vi "Initialize Network.vi"(8 "error in (no error)":errorcluster, 11 "msg cluster in":T1) -> (0 "error out":errorcluster, 2 "hardware controls out":T4={"force sensor channel"="", "servo task"="", "led task"="", "camera port"="", "cam freq (hz)"=30.0, "force freq (hz)"=30.0, "color pane"=0, "servo freq (hz)"=30.0} {"color pane" items=["Blue", "Red", "Green", "Saturation", "Value", "Intensity", "Luminance", "Hue", ""]}, 3 "msg cluster out":T1)   [LabVIEW 2020]
uses:
  Messaging Cluster.ctl
  Hardware/Sensors/Cameras/Camera.lvclass
  C:/Users/jharw/Documents/1 Folder to Rule them All/UMD/Inflation-Apparatus/src/Hardware/General Hardware.lvclass
  Hardware/Sensors/Force Sensors/Force Sensor.lvclass
  Hardware/Actuators/Servos/Servo.lvclass
  Hardware/Actuators/Switches/Switch.lvclass
  Inflation Test/Parameter Class/IA Test Parameters.lvclass
  Controllers/Controller.lvclass
  Controller Loop/Message and Data.ctl
  GUI/Main GUI Loop/Handler.ctl
  Inflation Test/Result Handling/Inflation Test Numeric Results.ctl
  Inflation Test/Controls/Hardware Options.ctl
  <vilib>/userdefined/High Color/IMAQdx.ctl
  Hardware/Sensors/Cameras/Simulated Camera/Simulated Camera.lvclass
  C:/Users/jharw/Documents/1 Folder to Rule them All/UMD/Inflation-Apparatus/src/Hardware/Sensors/Cameras/Camera.lvclass
  Hardware/Sensors/Force Sensors/Simulated Force Sensor/Simulated Force Sensor.lvclass
  C:/Users/jharw/Documents/1 Folder to Rule them All/UMD/Inflation-Apparatus/src/Hardware/Sensors/Force Sensors/Force Sensor.lvclass
  Hardware/Actuators/Servos/Simulated Servo/Simulated Servo.lvclass
  C:/Users/jharw/Documents/1 Folder to Rule them All/UMD/Inflation-Apparatus/src/Hardware/Actuators/Servos/Servo.lvclass
  Hardware/Actuators/Switches/Simulated Switch/Simulated Switch.lvclass
  C:/Users/jharw/Documents/1 Folder to Rule them All/UMD/Inflation-Apparatus/src/Hardware/Actuators/Switches/Switch.lvclass
  Hardware/General Hardware.lvclass/General Hardware.ctl
  Controllers/Simulated Controller/Simulated Controller.lvclass
  C:/Users/jharw/Documents/1 Folder to Rule them All/UMD/Inflation-Apparatus/src/Controllers/Controller.lvclass
  Controllers/PID/PID Controller.lvclass
  Controllers/PID/PID Controller.lvclass/PID Controller.ctl
  Hardware/General Hardware.lvclass
panel:
  in  "continue":bool
  in  "controller tab":enum32{"Simulated Controller", "PID Controller"}(tab)=enum."PID Controller"
  in  "PID gains":T6={"proportional gain (Kc)"=1.0, "integral time (Ti, min)"=0.01, "derivative time (Td, min)"=0.0} caption="PID GAINS" {"derivative time (Td, min)" format="%.3f"; "integral time (Ti, min)" format="%.3f"; "proportional gain (Kc)" format="%.3f"}
  in  "hardware tab":enum32{"Real Hardware", "Simulated Hardware"}(tab)
  in  "real hardware controls":T4={"force sensor channel"="", "servo task"="", "led task"="", "camera port"="", "cam freq (hz)"=30.0, "force freq (hz)"=30.0, "color pane"=0, "servo freq (hz)"=30.0} {"color pane" items=["Blue", "Red", "Green", "Saturation", "Value", "Intensity", "Luminance", "Hue", ""]}
  in  "sim servo freq (hz)":dbl=30.0
  in  "sim cam freq (hz)":dbl=30.0
  in  "sim force freq (hz)":dbl=30.0
  # "HARDWARE AND CONTROL INITIALIZATION"
  # "FORCE SENSOR CHANNEL"
  # "SERVO CHANNEL"
  # "LED CHANNEL"
  # "CAMERA PORT"
  # "CAMERA FREQUENCY (HZ):"
  # "FORCE FREQUENCY (HZ):"
  # "SERVO FREQUENCY (HZ):"
  # "COLOR PANE:"
  # "NO CONTROLLER WILL BE USED, GENERATED PULSES WILL BE RANDOM"
  # "FORCE SENSOR CHANNEL"
  # "SERVO CHANNEL"
  # "LED CHANNEL"
  # "CAMERA PORT"
  # "CAMERA FREQUENCY (HZ):"
  # "FORCE FREQUENCY (HZ):"
  # "SERVO FREQUENCY (HZ):"
  # "COLOR PANE:"
  # "CAMERA FREQUENCY (HZ):"
  # "FORCE FREQUENCY (HZ):"
  # "SERVO FREQUENCY (HZ):"
  # "CAMERA AND FORCE DATA GENERATED WILL BE RANDOMIZED\n\nSERVO AND LED WILL NOT INTERFACE WITH PHYSICAL HARDWARE"
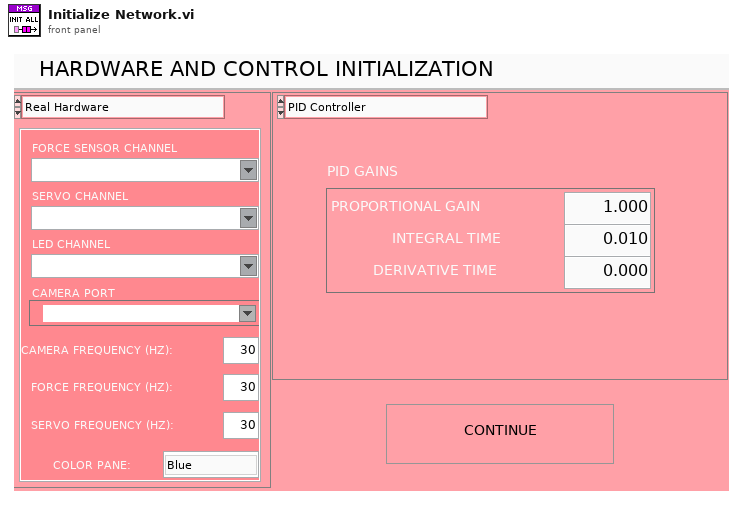
[diagram p1: front panel]
types:
  T1 = typedef "Messaging Cluster.ctl" = cluster{"cam queue":refnum<queue>, "fs queue":refnum<queue>, "servo queue":refnum<queue>, "switch queue":refnum<queue>, "cam class":refnum<class "Camera.lvclass">, "fs class":refnum<class "Force Sensor.lvclass">, "servo class":refnum<class "Servo.lvclass">, "switch class":refnum<class "Switch.lvclass">, "switch notifier":refnum<notifier>, "servo notifier":refnum<notifier>, "fs notifier":refnum<notifier>, "cam notifier":refnum<notifier>, "rgst evnt":refnum<event-registration>, "user event":refnum<user-event>, "ctlr queue":refnum<queue>, "main gui queue":refnum<queue>, "main gui type":T2, "cntlr type":T3, "gui notifier":refnum<notifier>, "ia test notifier":refnum<notifier>}
  T2 = typedef "Handler.ctl" = cluster{"bool ref":refnum<vi>, "error":errorcluster, "msg":string, "status":string}
  T3 = typedef "Message and Data.ctl" = cluster{"msg":string, "ia test param":refnum<class "IA Test Parameters.lvclass">, "controller type":refnum<class "Controller.lvclass">, "folder path":path, "file name":string, "file comments":string}
  T4 = typedef "Hardware Options.ctl" = cluster{"force sensor channel":tag, "servo task":tag, "led task":tag, "camera port":T5, "cam freq (hz)":dbl, "force freq (hz)":dbl, "color pane":i32, "servo freq (hz)":dbl}
  T5 = typedef "IMAQdx.ctl" = refnum<k21>
  T6 = cluster{"proportional gain (Kc)":dbl, "integral time (Ti, min)":dbl, "derivative time (Td, min)":dbl}
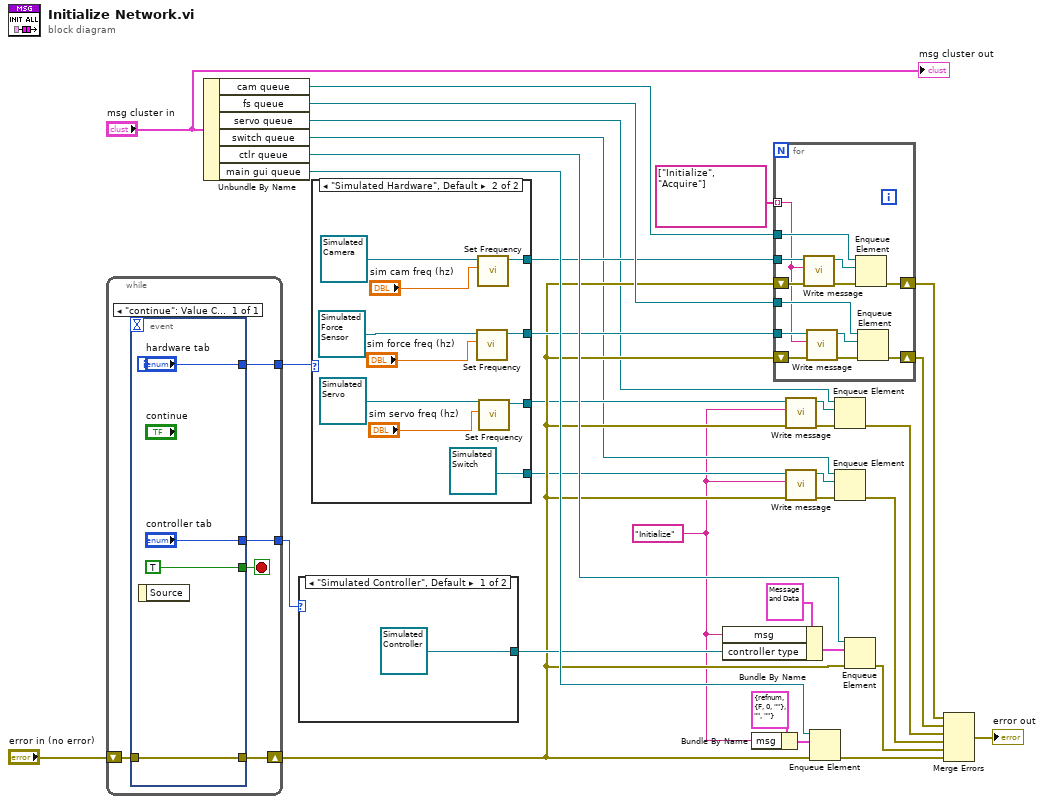
[diagram p0: block diagram]
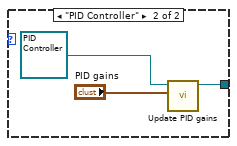
[diagram p2: hidden frame]
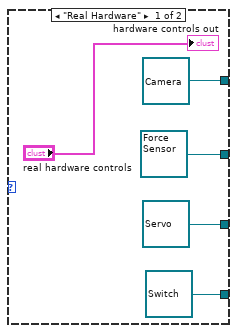
[diagram p3: hidden frame]
diagram:
  w4 = "Initialize" ("message")
  n1 = while {
    shift-right: [w37] -> w15
    shift-left: "error in (no error)" -> [w38]
    tunnel: [w35] -> w20
    tunnel: [w34] -> w17
    stop <- w36 stop-if-true
    n2 = event shown="[0] \"continue\": Value Change" {
      selector: _ -> [_]
      dyn-events: _ -> [_]
      timeout: _ -> [_]
      tunnel: w38 -> [w42]
      tunnel: [w42] -> w37
      tunnel: [TRUE] -> w36
      tunnel: ["hardware tab"] -> w35
      tunnel: ["controller tab"] -> w34
      event "continue": Value Change {
        n3 = event-data() -> ()  [unwired: 1 in, 1 out]
      }
    }
  }
  n4 = Unbundle By Name("msg cluster in") -> ("cam queue"=w3:refnum<queue>, "fs queue"=w32:refnum<queue>, "servo queue"=w9:refnum<queue>, "switch queue"=w8:refnum<queue>, "ctlr queue"=w31:refnum<queue>, "main gui queue"=w28:refnum<queue>)
  n5 = case shown="\"Simulated Controller\", Default" w17 {
    tunnel: [refnum<class "Simulated Controller.lvclass"> refnum ("Simulated Controller.lvclass") w44] -> w16
    frame "Simulated Controller", Default {
    }
    frame "PID Controller" {
      n6 = call "Update PID gains.vi"("PID gains"="PID gains", "PID Controller in"=refnum<class "PID Controller.lvclass"> refnum ("PID Controller.lvclass")) -> ("PID Controller out"=w44:refnum<class "PID Controller.lvclass">)  [unwired: 8 in, 1 out]
    }
  }
  n7 = case shown="\"Simulated Hardware\", Default" w20 {
    tunnel: [refnum<class "Camera.lvclass"> refnum ("Camera.lvclass") w57] -> w19
    tunnel: [refnum<class "Force Sensor.lvclass"> refnum ("Force Sensor.lvclass") w56] -> w18
    tunnel: [refnum<class "Servo.lvclass"> refnum ("Servo.lvclass") w54] -> w10
    tunnel: [refnum<class "Switch.lvclass"> refnum ("Switch.lvclass") refnum<class "Simulated Switch.lvclass"> refnum ("Simulated Switch.lvclass")] -> w11
    frame "Real Hardware" {
      "hardware controls out" <- "real hardware controls"
    }
    frame "Simulated Hardware", Default {
      n8 = call "Set Frequency.vi"("frequency (Hz)"="sim force freq (hz)", "General Hardware in"=refnum<class "Simulated Force Sensor.lvclass"> refnum ("Simulated Force Sensor.lvclass")) -> ("General Hardware out"=w56:refnum<class "Simulated Force Sensor.lvclass">)  [unwired: 8 in, 1 out]
      n9 = call "Set Frequency.vi"("frequency (Hz)"="sim cam freq (hz)", "General Hardware in"=refnum<class "Simulated Camera.lvclass"> refnum ("Simulated Camera.lvclass")) -> ("General Hardware out"=w57:refnum<class "Simulated Camera.lvclass">)  [unwired: 8 in, 1 out]
      n10 = call "Set Frequency.vi"("frequency (Hz)"="sim servo freq (hz)", "General Hardware in"=refnum<class "Simulated Servo.lvclass"> refnum ("Simulated Servo.lvclass")) -> ("General Hardware out"=w54:refnum<class "Simulated Servo.lvclass">)  [unwired: 8 in, 1 out]
    }
  }
  n11 = Bundle By Name(cluster=T3 {"msg"="", "ia test param"=refnum, "controller type"=refnum, "folder path"=path "", "file name"="", "file comments"=""} ("element"), "msg"=w4, "controller type"=w16) -> (w29:T3)
  n12 = Bundle By Name(cluster=T2 {"bool ref"=refnum, "error"={"status"=FALSE, "code"=0, "source"=""}, "msg"="", "status"=""} ("element"), "msg"=w4) -> (w26:T2)
  n13 = for {
    tunnel: w32 -> [w70]
    tunnel: w19 -> [w67]
    tunnel: w18 -> [w66]
    shift-right: [w69] -> w22
    shift-left: w15 -> [w68]
    shift-right: [w65] -> w2
    shift-left: w15 -> [w64]
    tunnel: w3 -> [w63]
    tunnel: string[] ["Initialize", "Acquire"] ("message") -> [w62] mode=indexing
    n14 = call "Write message.vi"("error in (no error)"=w68, "message"=w62, "General Hardware in"=w67) -> ("error out"=w73:errorcluster, "General Hardware out"=w74:refnum<class "Camera.lvclass">)  [unwired: 7 in]
    n15 = call "Write message.vi"("error in (no error)"=w64, "message"=w62, "General Hardware in"=w66) -> ("error out"=w72:errorcluster, "General Hardware out"=w71:refnum<class "Force Sensor.lvclass">)  [unwired: 7 in]
    n16 = Enqueue Element(queue=w63, element=w74, error in (no error)=w73) -> (error out=w69:errorcluster)  [unwired: 1 in, 2 out]
    n17 = Enqueue Element(queue=w70, element=w71, error in (no error)=w72) -> (error out=w65:errorcluster)  [unwired: 1 in, 2 out]
  }
  n18 = call "Write message.vi"("error in (no error)"=w15, "message"=w4, "General Hardware in"=w10) -> ("error out"=w12:errorcluster, "General Hardware out"=w14:refnum<class "Servo.lvclass">)  [unwired: 7 in]
  n19 = call "Write message.vi"("error in (no error)"=w15, "message"=w4, "General Hardware in"=w11) -> ("error out"=w5:errorcluster, "General Hardware out"=w13:refnum<class "Switch.lvclass">)  [unwired: 7 in]
  n20 = Enqueue Element(queue=w28, element=w26, error in (no error)=w15) -> (error out=w25:errorcluster)  [unwired: 1 in, 2 out]
  n21 = Enqueue Element(queue=w9, element=w14, error in (no error)=w12) -> (error out=w7:errorcluster)  [unwired: 1 in, 2 out]
  n22 = Enqueue Element(queue=w8, element=w13, error in (no error)=w5) -> (error out=w6:errorcluster)  [unwired: 1 in, 2 out]
  n23 = Enqueue Element(queue=w31, element=w29, error in (no error)=w15) -> (error out=w23:errorcluster)  [unwired: 1 in, 2 out]
  n24 = Merge Errors(w22, w2, w7, w6, w23, w25) -> (→"error out":errorcluster)
  "msg cluster out" <- "msg cluster in"
